vi "Read Output Till Keyword.vi"(7 "timeout [ms]":u32=1000, 8 "error in":errorcluster, 10 "keywords":string[](array[string])=["error", "USERkeyword"], 11 "GOLPI ref. in":T1={"pipe handle"={"lv_proc.dll file path"=path "", "process instance handle"=[], "debug mode"=FALSE, "debug data"=[]}, "fast read timeout [ms]"=500, "fast read settle time [ms]"=10, "fast read to multiple [ms]"=1, "max elements per input line"=100, "slow read timeout [ms]"=500, "stdin double format specifier"="", "max elements per stdout output column"=100, "console mode bitstream"=FALSE, "bitstream first read timeout [ms]"=1000, "bitstream read timeout [ms]"=50, "struct transfer possible"=FALSE, "matlab mode"=FALSE, "var pipe write timeout [ms]"=5000, "variable pipe mode"=FALSE, "variable pipe buffer size [Bytes]"=10000000, "variable pipe block size [Bytes]"=1000000} {"variable pipe block size [Bytes]" format="%.0p"; "variable pipe buffer size [Bytes]" format="%.0p"}) -> (0 "error out":errorcluster, 2 "read buffer":string, 3 "GOLPI ref. out":T1={"pipe handle"={"lv_proc.dll file path"=path "", "process instance handle"=[], "debug mode"=FALSE, "debug data"=[]}, "fast read timeout [ms]"=500, "fast read settle time [ms]"=10, "fast read to multiple [ms]"=1, "max elements per input line"=100, "slow read timeout [ms]"=500, "stdin double format specifier"="", "max elements per stdout output column"=100, "console mode bitstream"=FALSE, "bitstream first read timeout [ms]"=1000, "bitstream read timeout [ms]"=50, "struct transfer possible"=FALSE, "matlab mode"=FALSE, "var pipe write timeout [ms]"=5000, "variable pipe mode"=FALSE, "variable pipe buffer size [Bytes]"=10000000, "variable pipe block size [Bytes]"=1000000} {"variable pipe block size [Bytes]" format="%.0p"; "variable pipe buffer size [Bytes]" format="%.0p"}, 5 "bytes remaining":i32)   [LabVIEW 2020, in "GOLPI library.lvlib"]
doc: "Continually reads output of GNU Octave. If one of strings specified in keywords terminal is found in output, reading stops.\nIf timeout is exceeded, returns only part of buffer and returns number of bytes remaining in the stdout (if any).\nOne of keywords should be 'error' in the case error occurs, otherwise the vi will wait till timeout.\n\n---\nGOLPI works only with lv_proc.dll library, which is part of vipm package or should be delivered together with packed library. Placement of this dll is selected in terminal of Start GNU Octave.vi."
uses:
  GOLPI library.lvlib
  GOLPI reference Type Def.ctl
  LV Process source distribution/Pipe Handle.ctl
  Private/Type Definitions/Custom Error Codes Enum Type Def.vi
  LV Process source distribution/LV Process library.lvlib
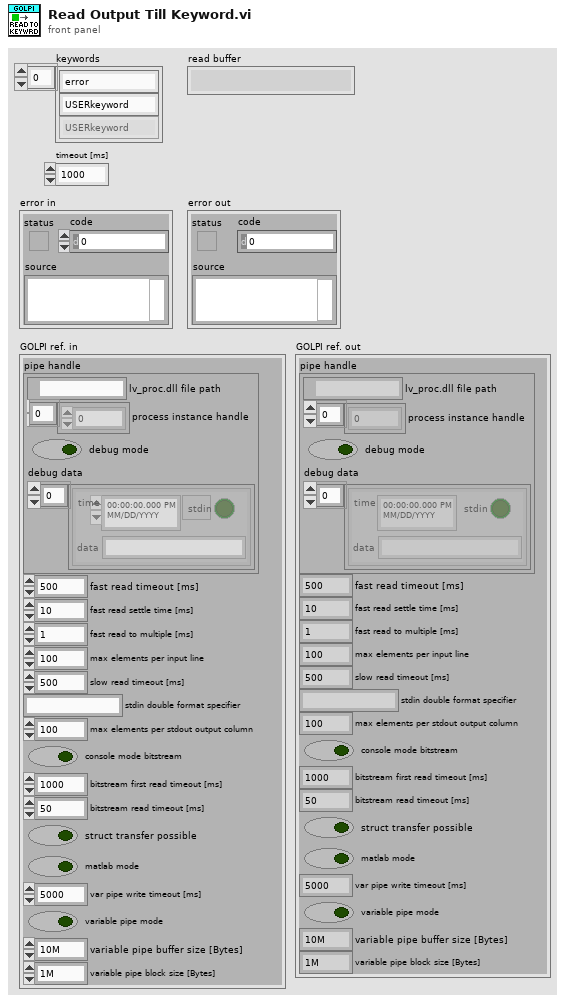
[diagram p1: front panel]
types:
  T1 = typedef "GOLPI library.lvlib/GOLPI reference Type Def.ctl" = cluster{"pipe handle":T2, "fast read timeout [ms]":u32, "fast read settle time [ms]":u32, "fast read to multiple [ms]":u32, "max elements per input line":u32, "slow read timeout [ms]":u32, "stdin double format specifier":string, "max elements per stdout output column":u32, "console mode bitstream":bool, "bitstream first read timeout [ms]":u32, "bitstream read timeout [ms]":u32, "struct transfer possible":bool, "matlab mode":bool, "var pipe write timeout [ms]":u32, "variable pipe mode":bool, "variable pipe buffer size [Bytes]":u32, "variable pipe block size [Bytes]":u32}
  T2 = typedef "LV Process library.lvlib/Pipe Handle.ctl" = cluster{"lv_proc.dll file path":path, "process instance handle":u32[], "debug mode":bool, "debug data":cluster{"time":timestamp, "stdin":bool, "data":string}[]}
  T3 = typedef "GOLPI library.lvlib/Custom Error Codes Enum Type Def.vi" = enum16{"no error", "00 working directory PAR1 missing", "01 octave binary PAR1 missing", "02 octave report error PAR1", "03 empty output last cmd PAR1", "04 missing temporary file PAR1", "05 pwd PAR 1 not exist", "06 oct package not installed", "07 octave default binary missing", "10 var PAR1 not string, vect", "11 var PAR1 not num, scal, ~compl", "12 var PAR1 not num, scal, compl", "13 var PAR1 not num, vect, ~compl", "14 var PAR1 not num, vect, compl", "15 var PAR1 not num, mat, ~compl", "16 var PAR1 not num, mat, ~compl", "30 read timeout", "60 bitstream transport failed", "61 bitstream decode error PAR1", "62 bitstream cannot be set", "70 struct transfer not possible", "80 struct: cluster elem. PAR1 not implem.", "81 struct: structure field PAR1 not implem.", "82 struct: size mismatch of PAR1", "83 struct: type mismatch of PAR1", "98 internal error", "99 not finished", "90 Not supported in Matlab mode", "91 Matlab variable transfer error", "92 Matlab Script Error"}
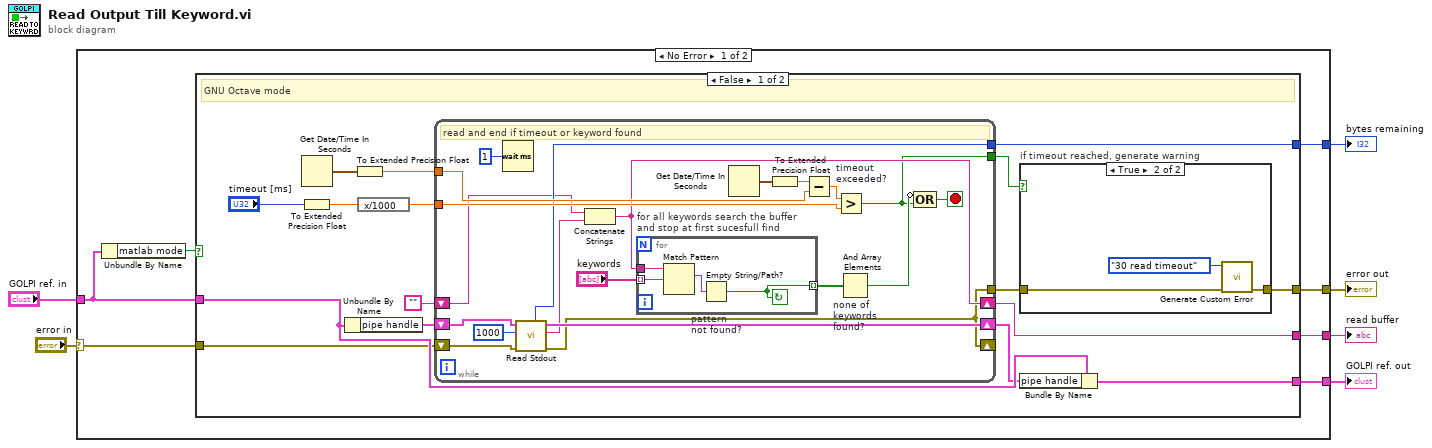
[diagram p0: block diagram]
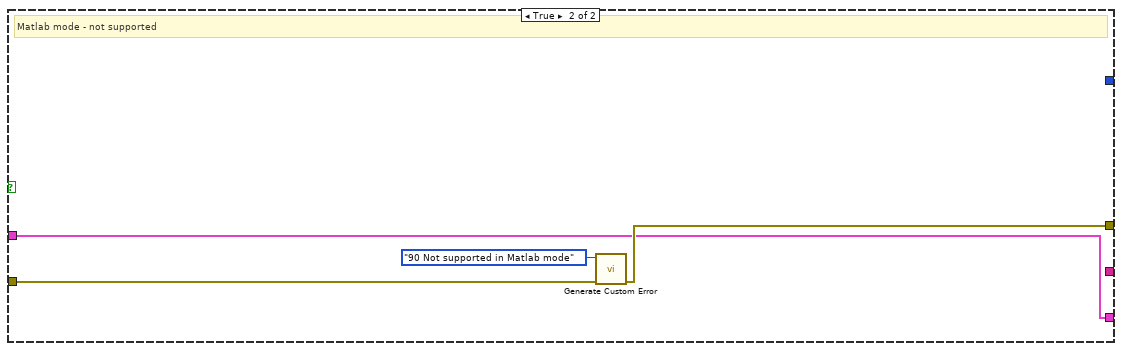
[diagram p3: hidden frame]
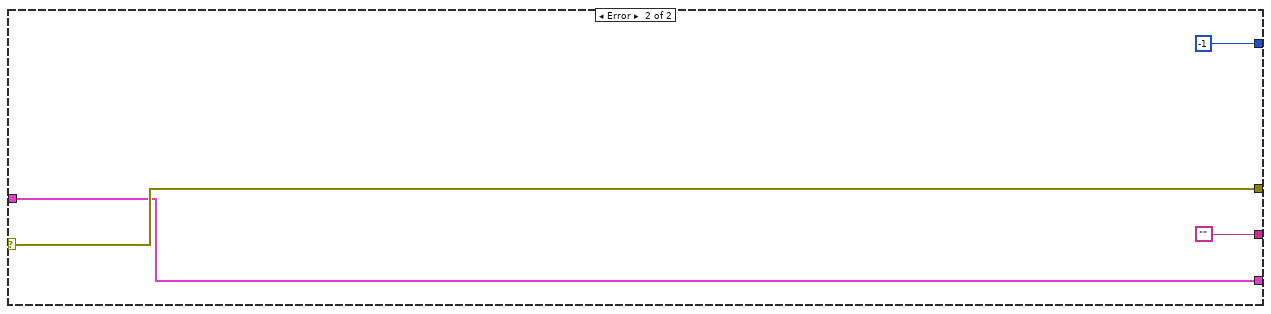
[diagram p4: hidden frame]
diagram:
  n1 = case shown="No Error" "error in" {
    selector: "error in" -> [w9 w65]
    tunnel: [w13 ""] -> w6
    tunnel: [w12 -1 ("bytes remaining")] -> w5
    tunnel: "GOLPI ref. in" -> [w8 w64]
    tunnel: [w11 w64] -> w3
    tunnel: [w10 w65] -> w2
    frame No Error {
      n2 = Unbundle By Name(w8) -> ("matlab mode"=w7:bool)
      n3 = case shown="False" w7 {
        tunnel: [w29 _] -> w13
        tunnel: [w28 _] -> w12
        tunnel: w8 -> [w26 w58]
        tunnel: [w25 w58] -> w11
        tunnel: [w21 w59] -> w10
        tunnel: w9 -> [w19 w61]
        frame False {
          # "GNU Octave mode"
          n4 = Get Date/Time In Seconds() -> (seconds since 1Jan1904=w18:timestamp)
          n5 = To Extended Precision Float(1:"timeout [ms]") -> (0:w15:ext)
          n6 = Unbundle By Name(w26) -> ("pipe handle"=w23:T2)
          n7 = To Extended Precision Float(1:w18) -> (0:w17:ext)
          n8 = expression code="x/1000"(w15) -> (w14:ext)
          n9 = while {
            tunnel: [w47] -> w28
            shift-right: [w52] -> w24
            shift-left: w23 -> [w53]
            shift-right: [w42] -> w29
            shift-left: "" -> [w43]
            tunnel: w17 -> [w50]
            tunnel: w14 -> [w48]
            shift-right: [w37] -> _
            shift-left: w19 -> [w51]
            tunnel: [w37] -> w22
            tunnel: [w36] -> w20
            stop <- w46 stop-if-true
            # "read and end if timeout or keyword found"
            n10 = Wait (ms)(milliseconds to wait=u32 1) -> ()  [unwired: 1 out]
            n11 = call "Read Stdout.vi"("error in"=w51, "byte count"=1000, "pipe in"=w53) -> ("error out"=w37:errorcluster, "read buffer"=w38:string, "pipe out"=w52:T2, "bytes remaining"=w47:i32)  [unwired: 3 in, 2 out]
            n12 = Concatenate Strings(w43, w38) -> (w42:string)
            n13 = for "for all keywords search the buffer\nand stop at first sucesfull find" {
              tunnel: w42 -> [w57]
              tunnel: "keywords" -> [w56] mode=indexing
              tunnel: [w54] -> w40 mode=indexing
              stop <- w54 continue-if-true
              n14 = Match Pattern(string=w57, regular expression=w56) -> (match substring=w55:string)  [unwired: 1 in, 3 out]
              n15 = Empty String/Path? "pattern\nnot found?"(string/path=w55) -> (empty?=w54:bool)
            }
            n16 = Get Date/Time In Seconds() -> (seconds since 1Jan1904=w35:timestamp)
            n17 = To Extended Precision Float(1:w35) -> (0:w34:ext)
            n18 = Subtract(x=w34, y=w50) -> (x-y=w49:ext)
            n19 = Greater? "timeout\nexceeded?"(x=w49, y=w48) -> (0:w36:bool)
            n20 = And Array Elements "none of\nkeywords\nfound?"(Boolean array=w40) -> (logical AND=w39:bool)
            n21 = Compound Arithmetic op=OR(invert w39, w36) -> (w46:bool)
          }
          n22 = case "if timeout reached, generate warning" shown="True" w20 {
            tunnel: [w30 w31] -> w21
            tunnel: w22 -> [w30 w32]
            frame False {
            }
            frame True {
              n23 = call "Generate Custom Error.vi"("error in"=w32, "GOLPI error"=Custom_Error_Codes_Enum_Type_Def.vi."30 read timeout") -> ("error out"=w31:errorcluster)  [unwired: 9 in]
            }
          }
          n24 = Bundle By Name(cluster=w26, "pipe handle"=w24) -> (w25:T1)
        }
        frame True {
          # "Matlab mode - not supported"
          n25 = call "Generate Custom Error.vi"("error in"=w61, "GOLPI error"=Custom_Error_Codes_Enum_Type_Def.vi."90 Not supported in Matlab mode") -> ("error out"=w59:errorcluster)  [unwired: 9 in]
        }
      }
    }
    frame Error {
    }
  }
  "error out" <- w2
  "read buffer" <- w6
  "bytes remaining" <- w5
  "GOLPI ref. out" <- w3
